vi "Query Correction.vi"(8 "error in (no error)":errorcluster, 9 "error message (f : no error)":bool, 11 "VISA resource name":refnum<visa-resource-name>) -> (0 "error out":errorcluster, 1 "correction on?":bool, 3 "VISA resource name out":refnum<visa-resource-name>)   [LabVIEW 2018, in "Agilent 87XX Series.lvlib"]
doc: "This VI for the HP8753B Network Analyzer is used to determine whether the correction is on or off. When the \"error message\" control is set to true, an error mesage will be generated in \"error out\" if correction is not on."
uses:
  Agilent 87XX Series.lvlib
panel:
  # "error message if correction off\nno error message"
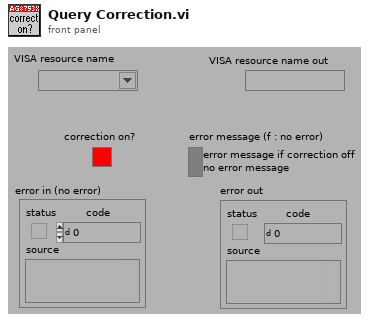
[diagram p1: front panel]
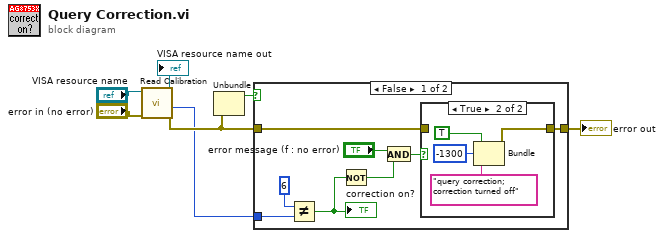
[diagram p0: block diagram]
diagram:
  n1 = call "Read Calibration.vi"("error in (no error)"="error in (no error)", "VISA resource name"="VISA resource name") -> ("error out"=w3:errorcluster, "cal type"=w2:i32, "VISA resource name out"=→"VISA resource name out":refnum<visa-resource-name>)  [unwired: 7 in]
  n2 = Unbundle(w3) -> ("status"=w4:bool)  [unwired: 2 out]
  n3 = case shown="False" w4 {
    tunnel: [w12 w21] -> w7
    tunnel: w3 -> [w11 w21]
    tunnel: w2 -> [w8 _]
    frame False {
      n4 = Not Equal?(x=6, y=w8) -> (x != y?=w10:bool)
      "correction on?" <- w10
      n5 = Not(x=w10) -> (.not. x?=w15:bool)
      n6 = And(x="error message (f : no error)", y=w15) -> (x .and. y?=w13:bool)
      n7 = case shown="True" w13 {
        tunnel: [w16 w17] -> w12
        tunnel: w11 -> [w16 _]
        frame False {
        }
        frame True {
          n8 = Bundle(TRUE, -1300, "query correction; correction turned off") -> (w17:errorcluster)  [unwired: 1 in]
        }
      }
    }
    frame True {
    }
  }
  "error out" <- w7
